vi "Write enemy_goalie_id.vi"(8 "error in (no error)":errorcluster, 10 "enemy_goalie_id":i32, 11 "Referee in":refnum<class "Referee.lvclass">) -> (0 "error out":errorcluster, 3 "Referee out":refnum<class "Referee.lvclass">)   [LabVIEW 2020, in "Referee.lvclass"]
uses:
  Referee.lvclass
  Referee.lvclass/Referee.ctl
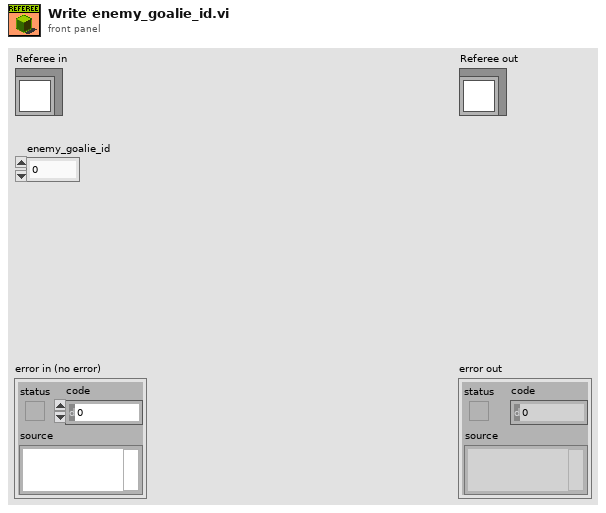
[diagram p1: front panel]
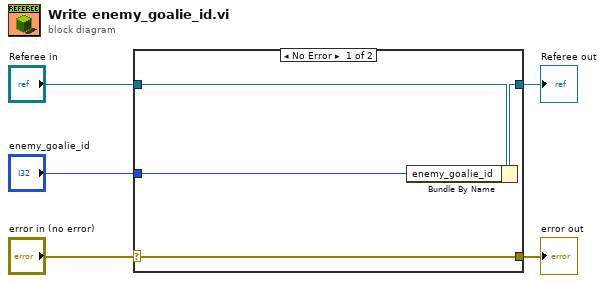
[diagram p0: block diagram]
diagram:
  n1 = case shown="No Error" "error in (no error)" {
    selector: "error in (no error)" -> [w9 w10]
    tunnel: [w9 w10] -> w4
    tunnel: [w7 w11] -> w2
    tunnel: "Referee in" -> [w8 w11]
    tunnel: "enemy_goalie_id" -> [w6 _]
    frame No Error {
      n2 = Bundle By Name(cluster=w8, "enemy_goalie_id"=w6) -> (w7:refnum<class "Referee.lvclass">)
    }
    frame Error {
    }
  }
  "error out" <- w4
  "Referee out" <- w2
